vi "CalGas aufschalten.vi"() -> (3 "Cluster":T1)   [LabVIEW 2020, in "Allgemein.lvlib"]
uses:
  Allgemein.lvlib
  FGV Analysator aktiv.ctl
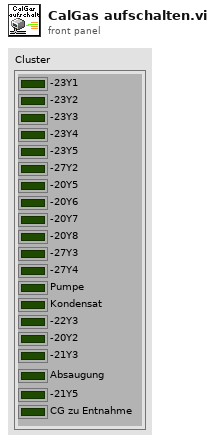
[diagram p1: front panel]
types:
  T1 = cluster{"-23Y1":bool, "-23Y2":bool, "-23Y3":bool, "-23Y4":bool, "-23Y5":bool, "-27Y2":bool, "-20Y5":bool, "-20Y6":bool, "-20Y7":bool, "-20Y8":bool, "-27Y3":bool, "-27Y4":bool, "Pumpe":bool, "Kondensat":bool, "-22Y3":bool, "-20Y2":bool, "-21Y3":bool, "Absaugung":bool, "-21Y5":bool, "CG zu Entnahme":bool}
  T2 = typedef "Allgemein.lvlib/FGV Analysator aktiv.ctl" = enum16{"lesen", "Analysator", "CG Aufschaltung", "KAL Zustand", "AutaKal GT?"}
  T3 = typedef "CalGas Aufschaltung.lvlib/Aufschaltung CalGas.ctl" = cluster{"Kalibriergas":T4, "Aufschaltpunkt":T5, "Analysator":T6}
  T4 = typedef "Auswahlfeld.ctl" = u16
  T5 = typedef "CalGas Aufschaltung.lvlib/Auswahl Aufschaltpunkt.ctl" = enum16{"über Filterblock", "Analysator direkt", "über PNS", "Entnahme", "Gasdivider"}
  T6 = typedef "CalGas Aufschaltung.lvlib/Auswahl Analysator.ctl" = enum16{"FT-IR", "FID", "PMA", "PMA/FID/FT-IR"}
  T7 = typedef "Status Analysatoren.lvlib/Status Analysatoren_Anzeige.ctl" = cluster{"FT-IR":bool, "FID":bool, "PMA":bool}
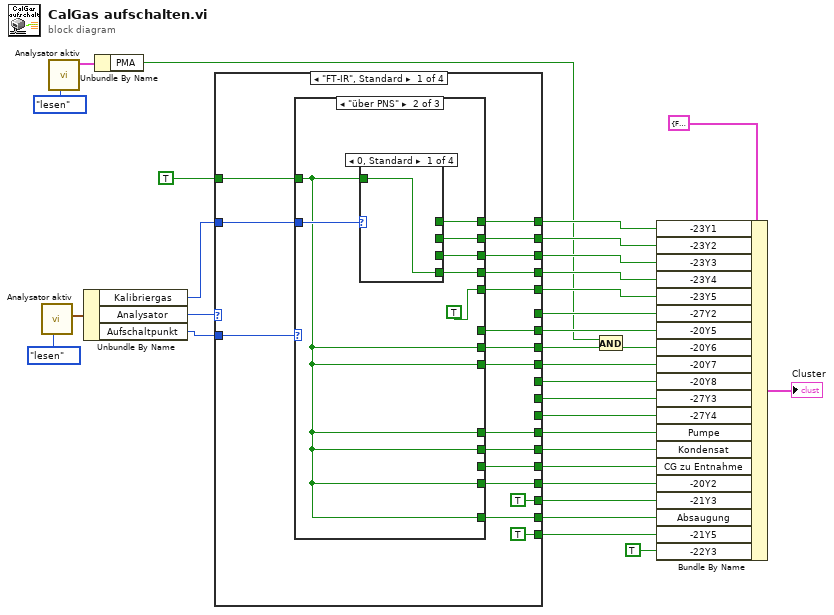
[diagram p0: block diagram]
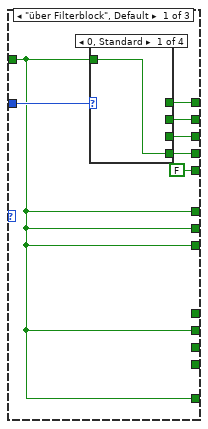
[diagram p2: hidden frame]
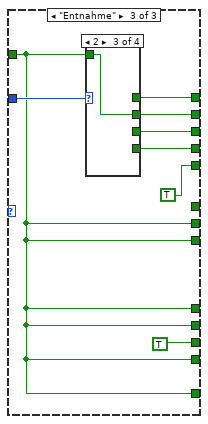
[diagram p9: hidden frame]
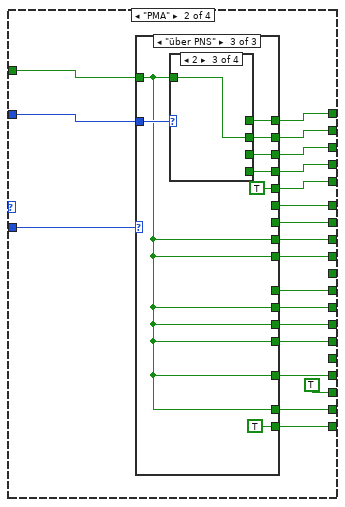
[diagram p13: hidden frame]
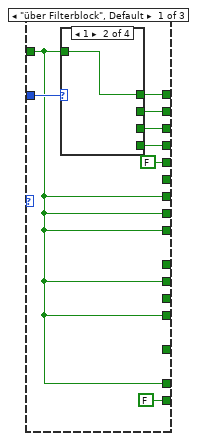
[diagram p14: hidden frame]
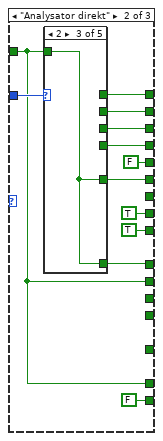
[diagram p18: hidden frame]
diagram:
  n1 = call "Analysator aktiv.vi"("Aktion"=FGV_Analysator_aktiv."lesen") -> ("Aufschaltung CalGas"=w31:T3)  [unwired: 7 in, 3 out]
  n2 = call "Analysator aktiv.vi"("Aktion"=FGV_Analysator_aktiv."lesen") -> ("Status Analysatoren"=w7:T7)  [unwired: 7 in, 3 out]
  n3 = Unbundle By Name(w31) -> ("Kalibriergas"=w13:T4, "Analysator"=w30:T6, "Aufschaltpunkt"=w29:T5)
  n4 = Unbundle By Name(w7) -> ("PMA"=w5:bool)
  n5 = case shown="\"FT-IR\", Standard" w30 {
    tunnel: w29 -> [w50 w104 w165 w212]
    tunnel: TRUE -> [w49 w103 w152 w199]
    tunnel: [w47 w101 w163 w210] -> w27
    tunnel: [w46 w100 w162 w209] -> w26
    tunnel: [w45 w99 w161 w208] -> w25
    tunnel: [w44 w98 w160 w207] -> w24
    tunnel: [w43 w97 w159 w206] -> w23
    tunnel: [_ w87 _ _] -> w22
    tunnel: [w42 w96 w158 w205] -> w21
    tunnel: [w35 w91 w148 w195] -> w20
    tunnel: [w41 w95 w157 w204] -> w19
    tunnel: [_ _ w154 w201] -> w18
    tunnel: [_ w88 _ _] -> w17
    tunnel: [_ w89 _ w192] -> w16
    tunnel: [w40 w94 w156 w203] -> w15
    tunnel: [w36 w90 w147 w194] -> w14
    tunnel: w13 -> [w48 w102 w164 w211]
    tunnel: [w39 w93 w155 w202] -> w12
    tunnel: [TRUE TRUE w150 w197] -> w11
    tunnel: [w37 w86 w149 w196] -> w10
    tunnel: [TRUE w85 TRUE TRUE] -> w9
    tunnel: [w33 _ _ _] -> w1
    frame "FT-IR", Default {
      n6 = case shown="\"über PNS\"" w50 {
        tunnel: w49 -> [w51 w62 w74]
        tunnel: w48 -> [w57 w68 w80]
        tunnel: [w56 w67 w79] -> w47
        tunnel: [w55 w66 w78] -> w46
        tunnel: [w54 w65 w77] -> w45
        tunnel: [w53 w64 w76] -> w44
        tunnel: [FALSE TRUE TRUE] -> w43
        tunnel: [w51 _ _] -> w42
        tunnel: [w51 w62 w74] -> w41
        tunnel: [_ w62 w74] -> w40
        tunnel: [_ w62 w74] -> w39
        tunnel: [w51 w62 w74] -> w37
        tunnel: [w51 w62 w74] -> w36
        tunnel: [w51 w62 w74] -> w35
        tunnel: [_ _ TRUE] -> w33
        frame "über Filterblock", Default {
          n7 = case shown="0, Standard" w57 {
            tunnel: w51 -> [w58 w59 w60 w61]
            tunnel: [_ w59 _ _] -> w56
            tunnel: [_ _ w60 _] -> w55
            tunnel: [_ _ _ w61] -> w54
            tunnel: [w58 _ _ _] -> w53
            frame 0, Default {
            }
            frame 1 {
            }
            frame 2 {
            }
            frame 3 {
            }
          }
        }
        frame "über PNS" {
          n8 = case shown="0, Standard" w68 {
            tunnel: w62 -> [w69 w70 w71 w72]
            tunnel: [_ w70 _ _] -> w67
            tunnel: [_ _ w71 _] -> w66
            tunnel: [_ _ _ w72] -> w65
            tunnel: [w69 _ _ _] -> w64
            frame 0, Default {
            }
            frame 1 {
            }
            frame 2 {
            }
            frame 3 {
            }
          }
        }
        frame "Entnahme" {
          n9 = case shown="2" w80 {
            tunnel: w74 -> [w81 w82 w83 w84]
            tunnel: [_ w82 _ _] -> w79
            tunnel: [_ _ w83 _] -> w78
            tunnel: [_ _ _ w84] -> w77
            tunnel: [w81 _ _ _] -> w76
            frame 0, Default {
            }
            frame 1 {
            }
            frame 2 {
            }
            frame 3 {
            }
          }
        }
      }
    }
    frame "PMA" {
      n10 = case shown="\"über PNS\"" w104 {
        tunnel: w103 -> [w106 w118 w135]
        tunnel: w102 -> [w112 w128 w141]
        tunnel: [w111 w127 w140] -> w101
        tunnel: [w110 w126 w139] -> w100
        tunnel: [w109 w125 w138] -> w99
        tunnel: [w108 w124 w137] -> w98
        tunnel: [FALSE FALSE TRUE] -> w97
        tunnel: [w106 _ _] -> w96
        tunnel: [w106 TRUE w135] -> w95
        tunnel: [_ _ w135] -> w94
        tunnel: [_ _ w135] -> w93
        tunnel: [w106 TRUE w135] -> w91
        tunnel: [w106 _ w135] -> w90
        tunnel: [w106 w118 w135] -> w89
        tunnel: [_ w121 _] -> w88
        tunnel: [_ w122 _] -> w87
        tunnel: [w106 w118 w135] -> w86
        tunnel: [FALSE FALSE TRUE] -> w85
        frame "über Filterblock", Default {
          n11 = case shown="1" w112 {
            tunnel: w106 -> [w113 w114 w115 w116]
            tunnel: [_ w114 _ _] -> w111
            tunnel: [_ _ w115 _] -> w110
            tunnel: [_ _ _ w116] -> w109
            tunnel: [w113 _ _ _] -> w108
            frame 0, Default {
            }
            frame 1 {
            }
            frame 2 {
            }
            frame 3 {
            }
          }
        }
        frame "Analysator direkt" {
          n12 = case shown="2" w128 {
            tunnel: w118 -> [w129 w130 w131 w132 w133]
            tunnel: [_ w130 _ _ _] -> w127
            tunnel: [_ _ _ _ w133] -> w126
            tunnel: [_ _ _ w132 _] -> w125
            tunnel: [w129 _ _ _ _] -> w124
            tunnel: [_ _ w131 _ _] -> w122
            tunnel: [_ _ w131 _ _] -> w121
            frame 0, Default {
            }
            frame 1 {
            }
            frame 2 {
            }
            frame 3 {
            }
            frame 4 {
            }
          }
        }
        frame "über PNS" {
          n13 = case shown="2" w141 {
            tunnel: w135 -> [w142 w143 w144 w145]
            tunnel: [_ w143 _ _] -> w140
            tunnel: [_ _ w144 _] -> w139
            tunnel: [_ _ _ w145] -> w138
            tunnel: [w142 _ _ _] -> w137
            frame 0, Default {
            }
            frame 1 {
            }
            frame 2 {
            }
            frame 3 {
            }
          }
        }
      }
    }
    frame "FID" {
      n14 = call "Verzoegerung.vi"("sec"=u16 12, "Startsignal"=w152) -> ("Zeit abgelaufen?"=w151:bool)  [unwired: 8 in, 1 out]
      n15 = case shown="\"über PNS\"" w165 {
        tunnel: w152 -> [w166 w179]
        tunnel: w164 -> [w174 w187]
        tunnel: [w173 w186] -> w163
        tunnel: [w172 w185] -> w162
        tunnel: [w171 w184] -> w161
        tunnel: [w170 w183] -> w160
        tunnel: [FALSE TRUE] -> w159
        tunnel: [w166 _] -> w158
        tunnel: [w166 w179] -> w157
        tunnel: [_ w179] -> w156
        tunnel: [_ w179] -> w155
        tunnel: [w168 w181] -> w154
        tunnel: w151 -> [w168 w181]
        tunnel: [w167 w180] -> w150
        tunnel: [w166 w179] -> w149
        tunnel: [w166 w179] -> w148
        tunnel: [w166 w179] -> w147
        frame "über Filterblock", Default {
          n16 = case shown="2" w174 {
            tunnel: w166 -> [w175 w176 w177 w178]
            tunnel: [_ w176 _ _] -> w173
            tunnel: [_ _ w177 _] -> w172
            tunnel: [_ _ _ w178] -> w171
            tunnel: [w175 _ _ _] -> w170
            frame 0, Default {
            }
            frame 1 {
            }
            frame 2 {
            }
            frame 3 {
            }
          }
          n17 = Not(x=w168) -> (.not. x?=w167:bool)
        }
        frame "über PNS" {
          n18 = case shown="2" w187 {
            tunnel: w179 -> [w188 w189 w190 w191]
            tunnel: [_ w189 _ _] -> w186
            tunnel: [_ _ w190 _] -> w185
            tunnel: [_ _ _ w191] -> w184
            tunnel: [w188 _ _ _] -> w183
            frame 0, Default {
            }
            frame 1 {
            }
            frame 2 {
            }
            frame 3 {
            }
          }
          n19 = Not(x=w181) -> (.not. x?=w180:bool)
        }
      }
    }
    frame "PMA/FID/FT-IR" {
      n20 = call "Verzoegerung.vi"("sec"=u16 12, "Startsignal"=w199) -> ("Zeit abgelaufen?"=w198:bool)  [unwired: 8 in, 1 out]
      n21 = case shown="\"über PNS\"" w212 {
        tunnel: w199 -> [w213 w227]
        tunnel: w211 -> [w221 w234]
        tunnel: [w220 w233] -> w210
        tunnel: [w219 w232] -> w209
        tunnel: [w218 w231] -> w208
        tunnel: [w217 w230] -> w207
        tunnel: [FALSE TRUE] -> w206
        tunnel: [w213 _] -> w205
        tunnel: [w213 w227] -> w204
        tunnel: [_ w227] -> w203
        tunnel: [_ w227] -> w202
        tunnel: [w215 w226] -> w201
        tunnel: w198 -> [w215 w226]
        tunnel: [w214 w228] -> w197
        tunnel: [w213 w227] -> w196
        tunnel: [w213 w227] -> w195
        tunnel: [w213 w227] -> w194
        tunnel: [w213 w226] -> w192
        frame "über Filterblock", Default {
          n22 = case shown="0, Standard" w221 {
            tunnel: w213 -> [w222 w223 w224 w225]
            tunnel: [_ w223 _ _] -> w220
            tunnel: [_ _ w224 _] -> w219
            tunnel: [_ _ _ w225] -> w218
            tunnel: [w222 _ _ _] -> w217
            frame 0, Default {
            }
            frame 1 {
            }
            frame 2 {
            }
            frame 3 {
            }
          }
          n23 = Not(x=w215) -> (.not. x?=w214:bool)
        }
        frame "über PNS" {
          n24 = case shown="1" w234 {
            tunnel: w227 -> [w235 w236 w237 w238]
            tunnel: [_ w236 _ _] -> w233
            tunnel: [_ _ w237 _] -> w232
            tunnel: [_ _ _ w238] -> w231
            tunnel: [w235 _ _ _] -> w230
            frame 0, Default {
            }
            frame 1 {
            }
            frame 2 {
            }
            frame 3 {
            }
          }
          n25 = Not(x=w226) -> (.not. x?=w228:bool)
        }
      }
    }
  }
  n26 = And(x=w5, y=w20) -> (x .and. y?=w6:bool)
  n27 = Bundle By Name(cluster=T1 {"-23Y1"=FALSE, "-23Y2"=FALSE, "-23Y3"=FALSE, "-23Y4"=FALSE, "-23Y5"=FALSE, "-27Y2"=FALSE, "-20Y5"=FALSE, "-20Y6"=FALSE, "-20Y7"=FALSE, "-20Y8"=FALSE, "-27Y3"=FALSE, "-27Y4"=FALSE, "Pumpe"=FALSE, "Kondensat"=FALSE, "-22Y3"=FALSE, "-20Y2"=FALSE, "-21Y3"=FALSE, "Absaugung"=FALSE, "-21Y5"=FALSE, "CG zu Entnahme"=FALSE} ("Cluster"), "-23Y1"=w27, "-23Y2"=w26, "-23Y3"=w25, "-23Y4"=w24, "-23Y5"=w23, "-27Y2"=w22, "-20Y5"=w21, "-20Y6"=w6, "-20Y7"=w19, "-20Y8"=w18, "-27Y3"=w17, "-27Y4"=w16, "Pumpe"=w15, "Kondensat"=w14, "CG zu Entnahme"=w1, "-20Y2"=w12, "-21Y3"=w11, "Absaugung"=w10, "-21Y5"=w9, "-22Y3"=TRUE) -> (→"Cluster":T1)
